vi "getMeasParams.vi"(0 "Matrix":T2) -> (4 "MeasParameters":T1 {"dsprsnSlope" format="%.2f"; "dispReferenceWL" format="%.2f"; "tdWinResBWGHz" format="%.2f"; "timeInc" format="%.2f"; "startFreq" format="%.2f"; "sampleSpacing" format="%.2f"; "avgDisp" format="%.2f"; "endWL" format="%.2f"; "dutLength" format="%.2f"}, 15 "error out":errorcluster)   [LabVIEW 2012]
uses:
  Matrices.ctl
  bin/OVA32.dll
panel:
  out "Output Value":i32
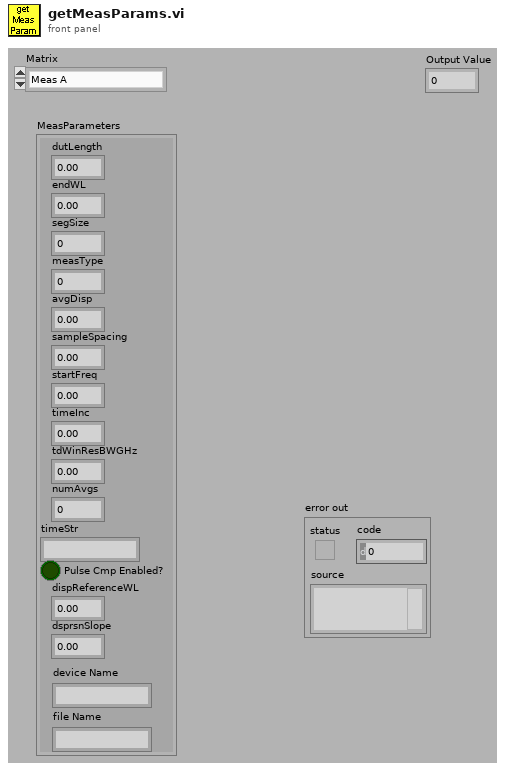
[diagram p1: front panel]
types:
  T1 = cluster{"dutLength":dbl, "endWL":dbl, "segSize":u32, "measType":u8, "avgDisp":dbl, "sampleSpacing":dbl, "startFreq":dbl, "timeInc":dbl, "tdWinResBWGHz":dbl, "numAvgs":u32, "timeStr":string, "Pulse Cmp Enabled?":bool, "dispReferenceWL":dbl, "dsprsnSlope":dbl, "device Name":string, "file Name":string}
  T2 = typedef "Matrices.ctl" = enum16{"Meas A", "Meas B", "Meas C", "Transfer", "Source", "Detector", "Temporary", "Temporary2", "Temporary3"}
  T3 = cluster{"dutLength":dbl, "endWL":dbl, "segSize":u32, "measType":u8, "avgDisp":dbl, "sampleSpacing":dbl, "startFreq":dbl, "timeInc":dbl, "tdResBwGHz":dbl, "numAvgs":u32, "timeStr":string, bool, "dispReferenceWL":dbl, "dsprsnSlope":dbl, "deviceDesciptor":string, "fileName":string}
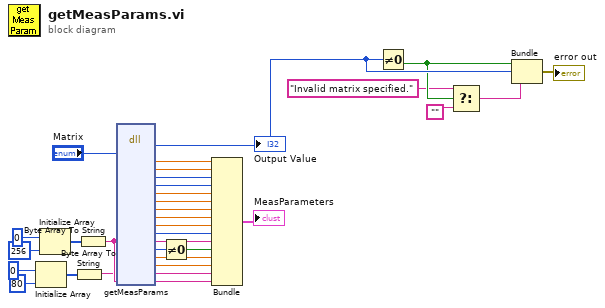
[diagram p0: block diagram]
diagram:
  n1 = Initialize Array(u8 0 ("Element Data"), 80 ("Dimension Size")) -> (w4:u8[])
  n2 = Initialize Array(u8 0 ("Element Data"), 256 ("Dimension Size")) -> (w25:u8[])
  n3 = Byte Array To String(unsigned byte array=w4) -> (string=w1:string)
  n4 = Byte Array To String(unsigned byte array=w25) -> (string=w5:string)
  n5 = dll-call lib="C:/_src/OVA5000_DSP_falcon/Software/LabVIEW/OVA/SDK/OVA_5000_SDK_v5.14.3/bin/OVA32.dll" fn="getMeasParams" label="getMeasParams()"("matrix"="Matrix", "timeStr"=w5, "deviceDesciptor"=w1, "fileName"=w5) -> (w20:i32, "dutLength"=w29:dbl, "endWL"=w30:dbl, "segSize"=w31:u32, "measType"=w32:u8, "avgDisp"=w24:dbl, "sampleSpacing"=w23:dbl, "startFreq"=w22:dbl, "timeInc"=w21:dbl, "tdResBwGHz"=w28:dbl, "numAvgs"=w13:u32, "timeStr"=w14:string, "cmpEnabled"=w10:u8, "dispReferenceWL"=w12:dbl, "dsprsnSlope"=w11:dbl, "deviceDesciptor"=w7:string, "fileName"=w6:string)  [unwired: 17 in, 2 out]
  "Output Value" <- w20
  n6 = Not Equal To 0?(x=w10) -> (x != 0?=w9:bool)
  n7 = Bundle("dutLength"=w29, "endWL"=w30, "segSize"=w31, "measType"=w32, "avgDisp"=w24, "sampleSpacing"=w23, "startFreq"=w22, "timeInc"=w21, "tdResBwGHz"=w28, "numAvgs"=w13, "timeStr"=w14, w9, "dispReferenceWL"=w12, "dsprsnSlope"=w11, "deviceDesciptor"=w7, "fileName"=w6) -> (→"MeasParameters":T3)  [unwired: 1 in]
  n8 = Not Equal To 0?(x=w20) -> (x != 0?=w18:bool)
  n9 = Select(t="Invalid matrix specified.", s=w18, f="") -> (s? t:f=w17:string)
  n10 = Bundle(w18, w20, w17) -> (→"error out":errorcluster)  [unwired: 1 in]
